vi "Configure Offset and Limits.vi"   [LabVIEW 2022 SP3, in "Agilent N934X Series.lvlib"]
doc: "This is a poly VI for Configure Offset and Limits VIs."
uses:
  <instrlib>/Agilent N934X Series/Agilent N934X Series.lvlib
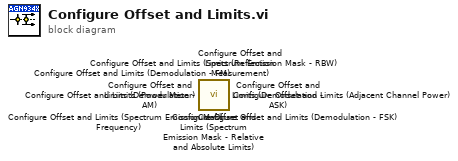
[diagram p0: block diagram]
diagram:
  n1 = call <instrlib>:"Configure Offset and Limits (Spectrum Emission Mask - Relative and Absolute Limits).vi"() -> ()  [unwired: 14 in, 2 out]
  n2 = call <instrlib>:"Configure Offset and Limits (Reflection Measurement).vi"() -> ()  [unwired: 14 in, 2 out]
  n3 = call <instrlib>:"Configure Offset and Limits (Demodulation - AM).vi"() -> ()  [unwired: 14 in, 2 out]
  n4 = call <instrlib>:"Configure Offset and Limits (Demodulation - ASK).vi"() -> ()  [unwired: 14 in, 2 out]
  n5 = call <instrlib>:"Configure Offset and Limits (Demodulation - FM).vi"() -> ()  [unwired: 14 in, 2 out]
  n6 = call <instrlib>:"Configure Offset and Limits (Demodulation - FSK).vi"() -> ()  [unwired: 14 in, 2 out]
  n7 = call <instrlib>:"Configure Offset and Limits (Spectrum Emission Mask - RBW).vi"() -> ()  [unwired: 14 in, 2 out]
  n8 = call <instrlib>:"Configure Offset and Limits (Spectrum Emission Mask - Frequency).vi"() -> ()  [unwired: 14 in, 2 out]
  n9 = call <instrlib>:"Configure Offset and Limits (Power Meter).vi"() -> ()  [unwired: 14 in, 2 out]
  n10 = call <instrlib>:"Configure Offset and Limits (Adjacent Channel Power).vi"() -> ()  [unwired: 14 in, 2 out]
